vi "eventStructure.vi"() -> ()   [LabVIEW 2025]
doc: "Uses the 'Value Change' event in LabVIEW to trigger actions when the value of a control or indicator changes."
uses:
  <vilib>/event_ctls.llb/lveventtype.ctl
panel:
  in  "Boolean 2":bool
  in  "stop":bool
  out "NewVal":bool
  out "OldVal":bool
  out "Type":T1=enum."Value Change"
  in  "Boolean":bool
  # "Events in Labview"
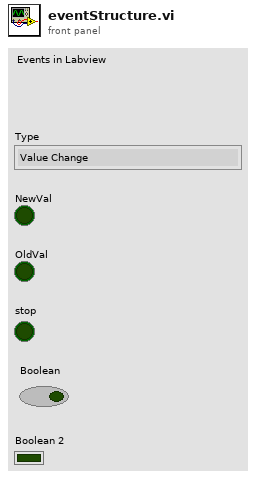
[diagram p1: front panel]
types:
  T1 = typedef "lveventtype.ctl" = enum32{"Null", "Timeout", "Annotation Menu Selection", "Annotation Menu Selection?", "App Instance Close", "App Instance Close?", "Autoscale Range Change", "Bookmark Info Change", "Cell Edit", "Cell Edit?", "Cursor Grab", "Cursor Grab?", "Cursor Menu Selection", "Cursor Menu Selection?", "Cursor Move", "Cursor Release", "Data Change", "Direction Change", "Display State Change", "Drag Ended", "Drag Enter", "Drag Leave", "Drag Over", "Drag Source Update", "Drag Starting", "Drag Starting?", "Drop", "Exec State Change", "Key Down", "Key Down?", "Key Repeat", "Key Repeat?", "Key Up", "Listbox Double Click", "Menu Activation?", "Menu Selection (App)", "Menu Selection? (App)", "Menu Selection (User)", "Mouse Down", "Mouse Down?", "Mouse Enter", "Mouse Leave", "Mouse Move", "Mouse Up", "Mouse Wheel", "NI Security User Change (App)", "Pane Size", "Panel Close", "Panel Close?", "Panel Resize", "Plot Attribute Change", "Scale Range Change", "Shortcut Menu Activation?", "Shortcut Menu Selection (App)", "Shortcut Menu Selection? (App)", "Shortcut Menu Selection (User)", "Tree Double Click", "Tree Drag", "Tree Drag?", "Tree Drop", "Tree Drop?", "Tree Item Close", "Tree Item Close?", "Tree Item Open", "Tree Item Open?", "User Event", "Value Change"}
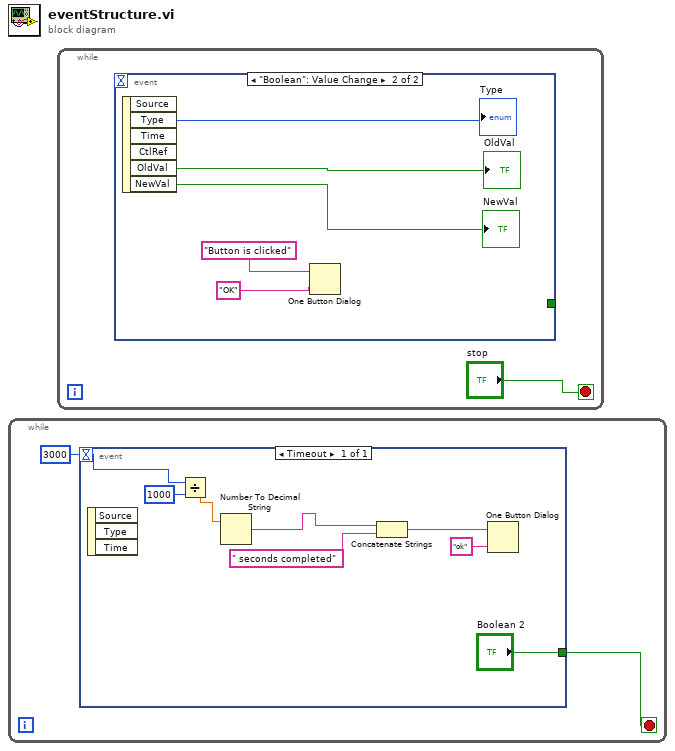
[diagram p0: block diagram]
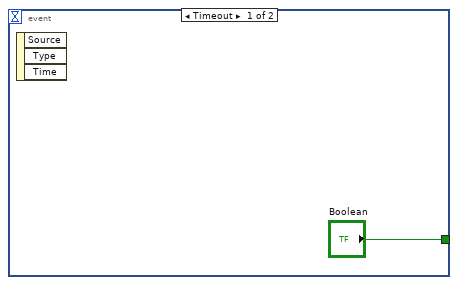
[diagram p2: hidden frame]
diagram:
  n1 = while {
    stop <- w1 stop-if-true
    n2 = event shown="[0] Timeout" {
      selector: _ -> [_]
      dyn-events: _ -> [_]
      timeout: 3000 -> [w10]
      tunnel: ["Boolean 2"] -> w1
      event Timeout {
        n3 = event-data() -> ()  [unwired: 1 in, 3 out]
        n4 = Divide(x=w10, y=1000) -> (x/y=w4:dbl)
        n5 = Number To Decimal String(number=w4) -> (decimal integer string=w3:string)  [unwired: 1 in]
        n6 = Concatenate Strings(w3, " seconds completed") -> (w7:string)
        n7 = One Button Dialog(message=w7, button name ("OK")="ok") -> ()  [unwired: 1 out]
      }
    }
  }
  n8 = while {
    stop <- "stop" stop-if-true
    n9 = event shown="[1] \"Boolean\": Value Change" {
      selector: _ -> [_ _]
      dyn-events: _ -> [_ _]
      timeout: _ -> [_ _]
      tunnel: ["Boolean" _] -> _
      event Timeout {
        n10 = event-data() -> ()  [unwired: 1 in, 3 out]
      }
      event "Boolean": Value Change {
        n11 = event-data() -> ("Type"=→"Type":T1, "OldVal"=→"OldVal":bool, "NewVal"=→"NewVal":bool)  [unwired: 1 in, 3 out]
        n12 = One Button Dialog(message="Button is clicked", button name ("OK")="OK") -> ()  [unwired: 1 out]
      }
    }
  }
